vi "MidBoxScanRepeatCheck.vi"(8 "error in":errorcluster caption="错误输入", 9 "StrIn":string, 11 "ArrayIn":string[](array[string])) -> (0 "error out":errorcluster caption="错误输出", 1 "StrOut":string, 3 "OK？":bool)   [LabVIEW 2013]
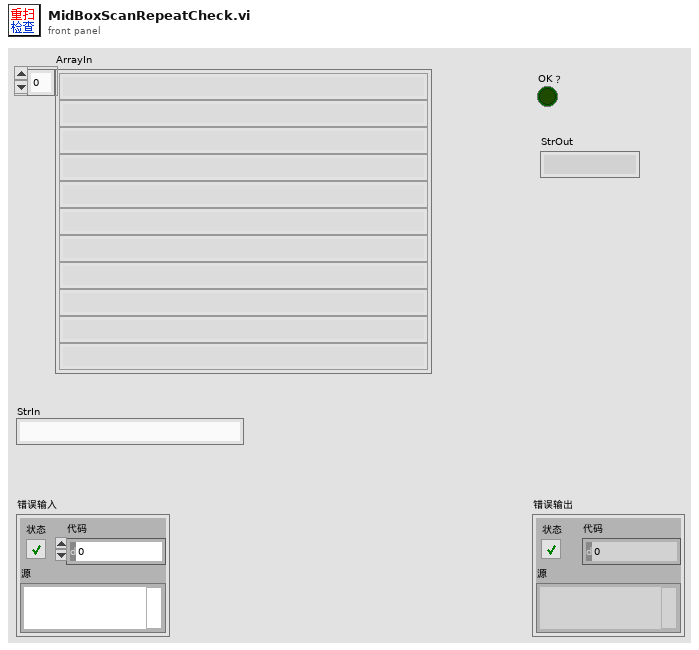
[diagram p1: front panel]
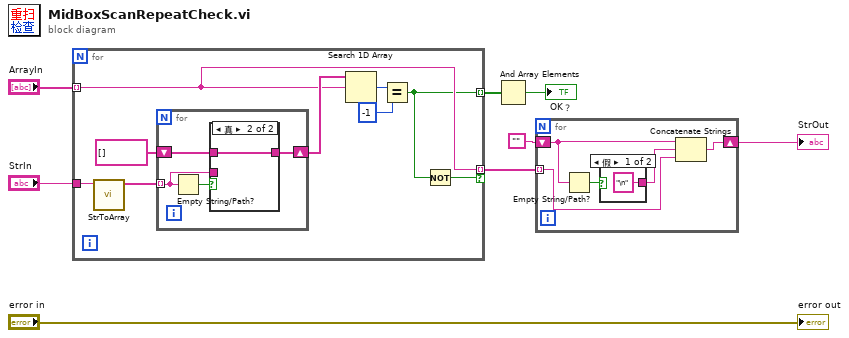
[diagram p0: block diagram]
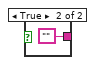
[diagram p2: hidden frame]
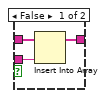
[diagram p3: hidden frame]
diagram:
  n1 = for {
    tunnel: "StrIn" -> [w17]
    tunnel: "ArrayIn" -> [w11] mode=indexing
    tunnel: [w9] -> w6 mode=indexing
    tunnel: [w11] -> w3 mode=indexing if=w10
    n2 = call "StrToArray.vi"("StrIn"=w17) -> ("ArrayOut"=w16:string[])  [unwired: 9 in, 1 out]
    n3 = for {
      tunnel: w16 -> [w19] mode=indexing
      shift-right: [w18] -> w14
      shift-left: string[] [] -> [w20]
      n4 = Empty String/Path?(string/path=w19) -> (empty?=w21:bool)
      n5 = case shown="真" w21 {
        tunnel: w20 -> [w24 w25]
        tunnel: w19 -> [w23 _]
        tunnel: [w22 w25] -> w18
        frame False {
          n6 = Insert Into Array(array=w24, new element=w23) -> (w22:string[])  [unwired: 1 in]
        }
        frame True {
        }
      }
    }
    n7 = Search 1D Array(1D array=w14, element=w11) -> (index of element=w13:i32)  [unwired: 1 in]
    n8 = Equal?(x=w13, y=-1) -> (x = y?=w9:bool)
    n9 = Not(x=w9) -> (.not. x?=w10:bool)
  }
  n10 = And Array Elements(Boolean array=w6) -> (logical AND=→"OK？":bool)
  n11 = for {
    shift-right: [w26] -> w2
    shift-left: "" -> [w30]
    tunnel: w3 -> [w27] mode=indexing
    n12 = Empty String/Path?(string/path=w30) -> (empty?=w29:bool)
    n13 = case shown="假" w29 {
      tunnel: ["\n" ""] -> w28
      frame False {
      }
      frame True {
      }
    }
    n14 = Concatenate Strings(w30, w28, w27) -> (w26:string)
  }
  "StrOut" <- w2
  "error out" <- "error in"
